vi "_API_BINANCE_GET_trades.vi"(0 "BinanceAPI in":refnum<class "BinanceAPI_.lvclass">, 5 "Depth":T2, 11 "error in (no error)":errorcluster) -> (4 "BinanceAPI out":refnum<class "BinanceAPI_.lvclass">, 6 "data":T1(array[cluster]), 14 "Data":string, 15 "error out":errorcluster)   [LabVIEW 2022 SP3, in "BinanceAPI_.lvclass"]
doc: "https://binance-docs.github.io/apidocs/spot/en/#recent-trades-list"
uses:
  BinanceAPI_.lvclass
  BinanceAPI_.lvclass/BinanceAPI_.ctl
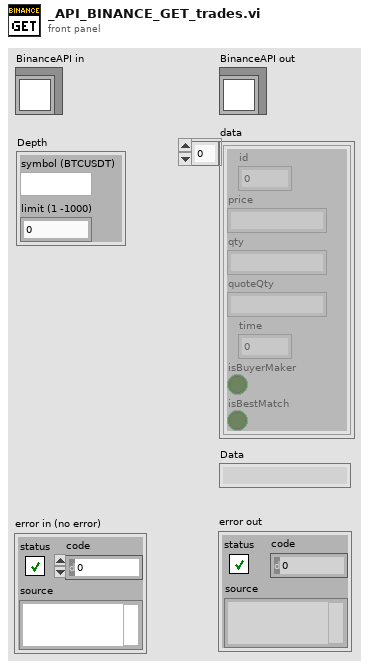
[diagram p1: front panel]
types:
  T1 = cluster{"id":dbl, "price":string, "qty":string, "quoteQty":string, "time":dbl, "isBuyerMaker":bool, "isBestMatch":bool}[]
  T2 = cluster{"symbol (BTCUSDT)":string, "limit (1 -1000)":i16}
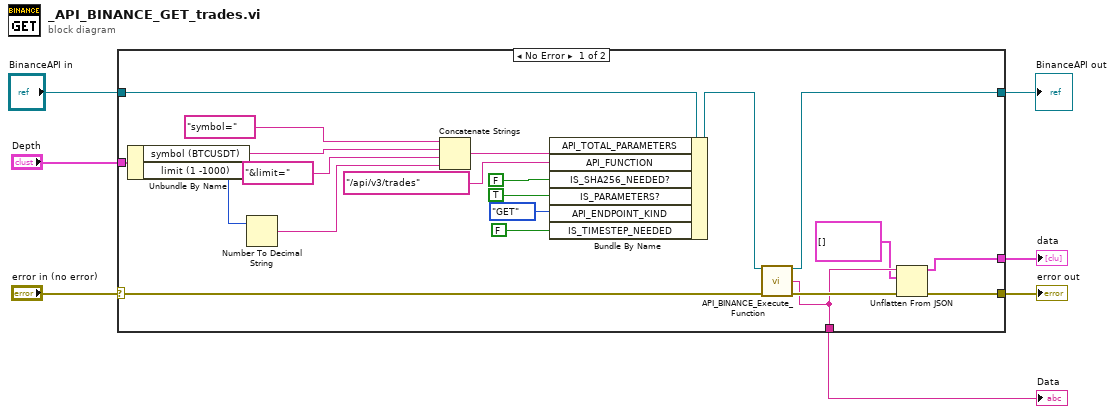
[diagram p0: block diagram]
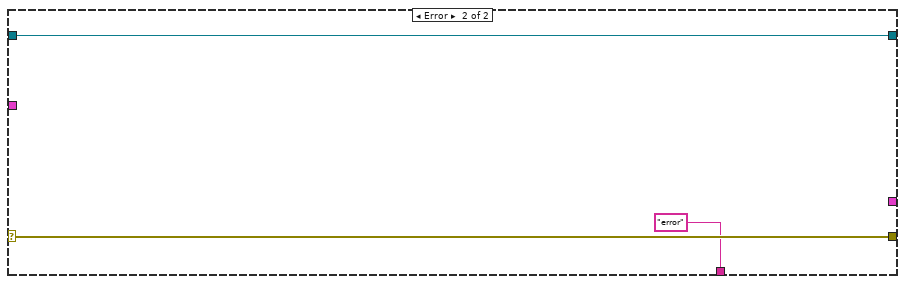
[diagram p2: hidden frame]
diagram:
  n1 = case shown="No Error" "error in (no error)" {
    selector: "error in (no error)" -> [w16 w31]
    tunnel: [w11 w31] -> w5
    tunnel: [w17 w30] -> w2
    tunnel: "BinanceAPI in" -> [w28 w30]
    tunnel: "Depth" -> [w21 _]
    tunnel: [w10 "error" ("Dane")] -> w4
    tunnel: [w9 _] -> w3
    frame No Error {
      n2 = Unbundle By Name(w21) -> ("symbol (BTCUSDT)"=w20:string, "limit (1 -1000)"=w14:i16)
      n3 = Number To Decimal String(number=w14) -> (decimal integer string=w13:string)  [unwired: 1 in]
      n4 = Concatenate Strings("symbol=", w20, "&limit=", w13) -> (w22:string)
      n5 = Bundle By Name(cluster=w28, "API_TOTAL_PARAMETERS"=w22, "API_FUNCTION"="/api/v3/trades", "IS_SHA256_NEEDED?"=FALSE, "IS_PARAMETERS?"=TRUE, "API_ENDPOINT_KIND"=enum16{"POST", "DELETE", "GET", "PUT"}."GET", "IS_TIMESTEP_NEEDED"=FALSE) -> (w18:refnum<class "BinanceAPI_.lvclass">)
      n6 = call "API_BINANCE_Execute_Function.vi"("BinanceAPI in"=w18, "error in (no error)"=w16) -> ("BinanceAPI out"=w17:refnum<class "BinanceAPI_.lvclass">, "Body"=w10:string, "error out"=w12:errorcluster)  [unwired: 9 in, 2 out]
      n7 = Unflatten From JSON(JSON string=w10, type and defaults=T1 [], error in (no error)=w12) -> (value=w9:T1, error out=w11:errorcluster)  [unwired: 4 in]
    }
    frame Error {
    }
  }
  "error out" <- w5
  "Data" <- w4
  "data" <- w3
  "BinanceAPI out" <- w2
